vi "MDPtr Get Info.vi"(10 "error in (no error)":errorcluster, 11 "HexStrPtr":T1) -> (0 "Copy Count":i32, 1 "Data Type":T2, 2 "error out":errorcluster, 3 "HexStrPtr (dup)":T1, 4 "String Attribute":string)   [LabVIEW 2014]
uses:
  MDPtr TypeDef/MDPtr.ctl
  MDPtr TypeDef/MDPtr SupportedDataTypeDef.ctl
  MDPtr TypeDef/MDPtr DataFrame-Common.ctl
  <userlib>/_OpenG.lib/error/error.llb/Build Error Cluster__ogtk.vi
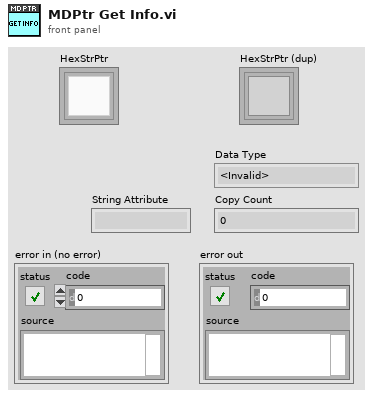
[diagram p1: front panel]
types:
  T1 = typedef "MDPtr.ctl" = refnum<k1>
  T2 = typedef "MDPtr SupportedDataTypeDef.ctl" = enum16{"<Invalid>", "Waveform", "Waveform Arr", "Double Arr", "String Arr"}
  T3 = typedef "MDPtr DataFrame-Common.ctl" = cluster{"Data Type":T2, "Copy Count":i32, "String Attribute":string}
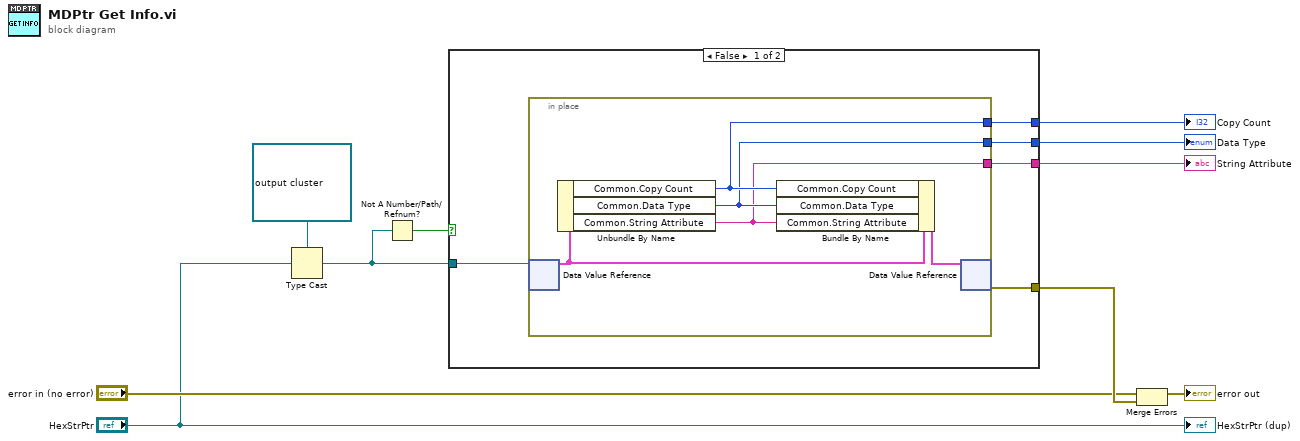
[diagram p0: block diagram]
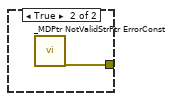
[diagram p2: hidden frame]
diagram:
  n1 = Type Cast(type=refnum<data-value> refnum ("data value reference"), x="HexStrPtr") -> (*(type *) &x=w3:refnum<data-value>)
  n2 = Not A Number/Path/Refnum?(number/path/refnum=w3) -> (NaN/Path/Refnum?=w2:bool)
  n3 = case shown="False" w2 {
    tunnel: [w15 w21] -> w10
    tunnel: w3 -> [w14 _]
    tunnel: [w13 _] -> w7
    tunnel: [w12 _] -> w6
    tunnel: [w11 _] -> w1
    frame False {
      n4 = in-place {
        in-place-border: [w18] -> w13
        in-place-border: [w17] -> w12
        in-place-border: [w16] -> w11
        n5 = in-place-dvr #1(w14) -> (w20:cluster{"Common":T3})  [unwired: 1 out]
        n6 = Unbundle By Name(w20) -> ("Common.Copy Count"=w18:i32, "Common.Data Type"=w17:T2, "Common.String Attribute"=w16:string)
        n7 = Bundle By Name(cluster=w20, "Common.Copy Count"=w18, "Common.Data Type"=w17, "Common.String Attribute"=w16) -> (w19:cluster{"Common":T3})
        n8 = in-place-dvr #1(w19) -> (w15:errorcluster)  [unwired: 1 out]
      }
    }
    frame True {
      n9 = call "_MDPtr NotValidStrPtr ErrorConst.vi"() -> ("error out"=w21:errorcluster)  [unwired: 19 in]
    }
  }
  "Copy Count" <- w7
  "Data Type" <- w6
  "String Attribute" <- w1
  n10 = Merge Errors("error in (no error)", w10) -> (→"error out":errorcluster)
  "HexStrPtr (dup)" <- "HexStrPtr"
